vi "Coord window-Request bring to front.vi"(8 "error in (no error)":errorcluster) -> (0 "error out":errorcluster)   [LabVIEW 2017]
uses:
  Globals/Coord window-Globals.vi
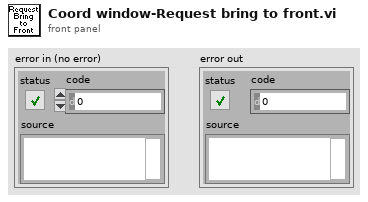
[diagram p1: front panel]
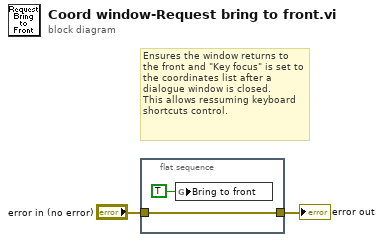
[diagram p0: block diagram]
diagram:
  # "Ensures the window returns to the front and \"Key focus\" is set to the coordinates list after a dialogue window is closed.\nThis allows ressuming keyboard shortcuts control."
  n1 = flat-sequence {
    tunnel: "error in (no error)" -> [w3]
    tunnel: [w3] -> w2
    frame #0 {
      n2 = global write "Coord window-Globals.vi" "Bring to front"(TRUE ("Bring to front")) -> ()
    }
  }
  "error out" <- w2
